vi "Read TestStatus.vi"(11 "Logger in":refnum<class "TestDataLog.lvclass">) -> (2 "TestStatus":T1 {"demandedProfileSteps" min=1; "demandedCycles" min=1; "activeProfileStep" min=1; "activeCycle" min=1}, 3 "Logger out":refnum<class "TestDataLog.lvclass">)   [LabVIEW 2015]
uses:
  TestDataLog.lvclass
  Typedefs/TestStatus.ctl
  Typedefs/M1M3SSSTypedefs.lvlib
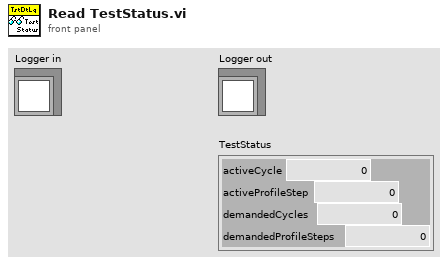
[diagram p1: front panel]
types:
  T1 = typedef "M1M3SSSTypedefs.lvlib/TestStatus.ctl" = cluster{"activeCycle":u32, "activeProfileStep":u32, "demandedCycles":u32, "demandedProfileSteps":u32}
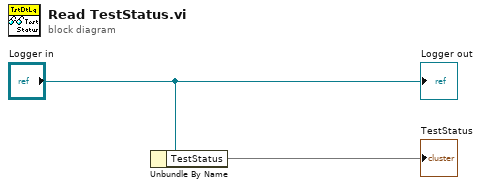
[diagram p0: block diagram]
diagram:
  n1 = Unbundle By Name("Logger in") -> ("TestStatus"=→"TestStatus")
  "Logger out" <- "Logger in"
